vi "Merge JSON.vi"(8 "error in (no error)":errorcluster, 10 "<JSON> to merge in":string="{\n    \"properties\":{\n         \"Module\":{\"description\":\"This is a legacy parameter, kept as optional for compatability\",\"type\":\"string\"}\n      },\n     \"description\": \"This schema describes the parameters of the Trigger Subsystem\",\n\"test\":\"new attribute\"\n\n}", 11 "<JSON> in":string="{\n    \"description\": \"This is a cluster\",\n    \"type\": \"object\",\n     \"required\": [\"Trigger Timeout (ms)\",\"Trigger Pulse Duration (s)\",\"Trigger Samplerate (Hz)\",\"Triggers\"],\n     \"properties\": {\"Trigger Timeout (ms)\":{\"description\":\"\",\"type\":\"integer\"},\"Trigger Pulse Duration (s)\":{\"description\":\"\",\"type\":\"number\"},\"Trigger Samplerate (Hz)\":{\"description\":\"\",\"type\":\"number\"},\"Triggers\":{\"description\":\"Setup the required Triggers\",\"type\":\"array\",\"default\":{\n        \"Channel\":\"No Trigger\",\n        \"Settings\":{\"Delay (s)\":0,\"Main Trigger?\":false}\n      },\"uniqueItems\":true,\"items\":{\"description\":\"\",\"type\":\"object\",\"required\":[\"Channel\",\"Settings\"],\"properties\":{\"Channel\":{\"$ref\":\"#/$defs/nova-subsystems-shared.lvlib:Trigger_Channels--enum.ctl\"},\"Settings\":{\"description\":\"\",\"type\":\"object\",\"required\":[\"Delay (s)\",\"Main Trigger?\"],\"properties\":{\"Delay (s)\":{\"description\":\"\",\"type\":\"number\"},\"Main Trigger?\":{\"description\":\"\",\"type\":\"boolean\"}}}}}}}\n}") -> (0 "error out":errorcluster, 3 "<JSON> out":string caption="<JSON>Merged")   [LabVIEW 2020, in "JSON Schema Generator.lvlib"]
uses:
  JSON Schema Generator.lvlib
  <vilib>/JDP Science/JSONtext/JSONtext.lvlib
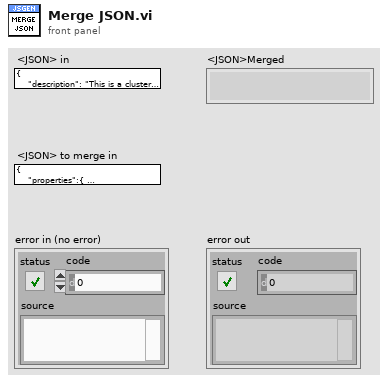
[diagram p1: front panel]
types:
  T1 = typedef "JSONtext.lvlib/JSON Value Type.ctl" = enum16{"Not a JSON Value", "JSON Object", "JSON Array", "String", "Number", "true", "false", "null"}
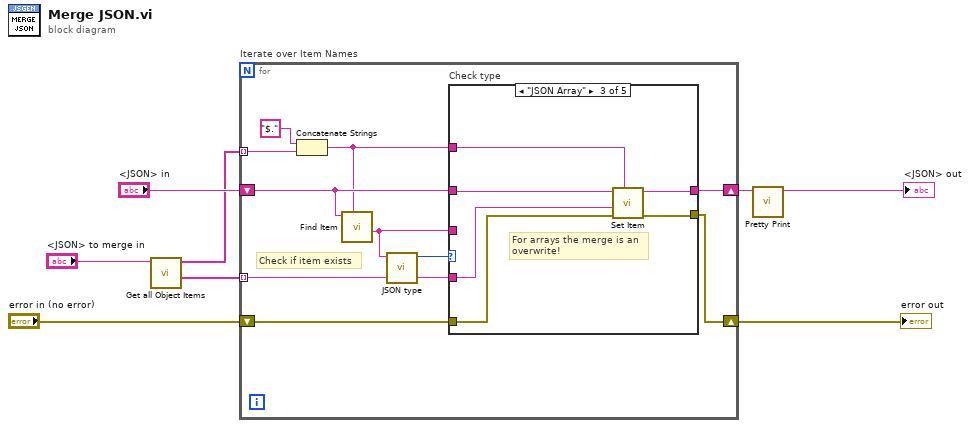
[diagram p0: block diagram]
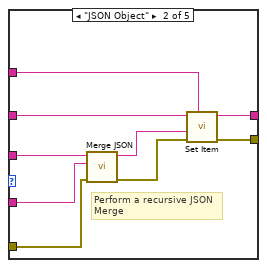
[diagram p3: hidden frame]
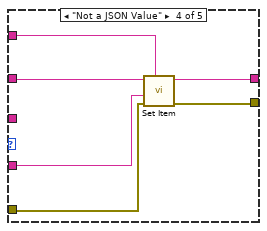
[diagram p4: hidden frame]
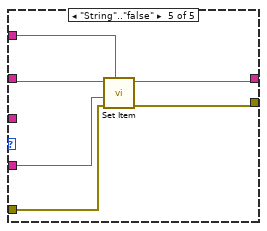
[diagram p5: hidden frame]
diagram:
  n1 = call <vilib>:"Get all Object Items.vi"("JSON"="<JSON> to merge in") -> ("<JSON>"=w4:string[], "Item Names"=w5:string[])  [unwired: 7 in, 2 out]
  n2 = for "Iterate over Item Names" {
    tunnel: w5 -> [w16] mode=indexing
    shift-right: [w18] -> w7
    shift-left: "<JSON> in" -> [w14]
    tunnel: w4 -> [w13] mode=indexing
    shift-right: [w15] -> w2
    shift-left: "error in (no error)" -> [w9]
    # "Check if item exists"
    n3 = Concatenate Strings("$." ("string"), w16) -> (w12:string)
    n4 = call <vilib>:"Find Item.vi"("$Path or Item Name"=w12, "JSON"=w14) -> ("<JSON>"=w10:string)  [unwired: 6 in, 3 out]
    n5 = call <vilib>:"JSON type.vi"("JSON"=w10) -> ("JSON Value Type"=w11:T1)  [unwired: 9 in, 1 out]
    n6 = case "Check type" shown="\"JSON Array\"" w11 {
      tunnel: [w20 w29 w33 w39 w44] -> w18
      tunnel: w12 -> [_ w28 w32 w38 w46]
      tunnel: [w19 w27 w35 w37 w43] -> w15
      tunnel: w14 -> [w20 w26 w34 w41 w47]
      tunnel: w13 -> [_ w23 w30 w40 w45]
      tunnel: w10 -> [_ w25 _ _ _]
      tunnel: w9 -> [w19 w21 w31 w36 w42]
      frame "null" {
      }
      frame "JSON Object" {
        # "Perform a recursive JSON\nMerge"
        n7 = call "Merge JSON.vi"("error in (no error)"=w21, "<JSON> to merge in"=w23, "<JSON> in"=w25) -> ("error out"=w22:errorcluster, "<JSON> out"=w24:string)  [unwired: 7 in]
        n8 = call <vilib>:"Set Item.vi"("$Path or Item Name"=w28, "error in (no error)"=w22, "JSON to Insert"=w24, "JSON"=w26) -> ("error out"=w27:errorcluster, "<JSON>"=w29:string)  [unwired: 4 in, 1 out]
      }
      frame "JSON Array" {
        # "For arrays the merge is an \noverwrite!"
        n9 = call <vilib>:"Set Item.vi"("$Path or Item Name"=w32, "error in (no error)"=w31, "JSON to Insert"=w30, "JSON"=w34) -> ("error out"=w35:errorcluster, "<JSON>"=w33:string)  [unwired: 4 in, 1 out]
      }
      frame "Not a JSON Value" {
        n10 = call <vilib>:"Set Item.vi"("$Path or Item Name"=w38, "error in (no error)"=w36, "JSON to Insert"=w40, "JSON"=w41) -> ("error out"=w37:errorcluster, "<JSON>"=w39:string)  [unwired: 4 in, 1 out]
      }
      frame "String".."false" {
        n11 = call <vilib>:"Set Item.vi"("$Path or Item Name"=w46, "error in (no error)"=w42, "JSON to Insert"=w45, "JSON"=w47) -> ("error out"=w43:errorcluster, "<JSON>"=w44:string)  [unwired: 4 in, 1 out]
      }
    }
  }
  "error out" <- w2
  n12 = call <vilib>:"Pretty Print.vi"("JSON"=w7) -> ("<JSON>"=→"<JSON> out":string)  [unwired: 8 in, 2 out]
